vi "SimplePassRollRole.vi"(6 "Tactic index in":i32, 7 "first call":bool, 8 "error in (no error)":errorcluster, 10 "Game in":refnum<class "Game.lvclass">, 11 "SimplePassRollRole in":refnum<class "SimplePassRollRole.lvclass">) -> (0 "error out":errorcluster, 1 "tactic index":i32, 2 "Robot out":refnum<class "Robot.lvclass">, 3 "SimplePassRollRole out":refnum<class "SimplePassRollRole.lvclass">)   [LabVIEW 2023, in "SimplePassRollRole.lvclass"]
uses:
  SimplePassRollRole.lvclass
  Game_class/Game.lvclass
  Robot_class/Robot.lvclass
  Role_class/Role.lvclass/Role.ctl
  Tacticbook_class/Tacticbook.lvclass/Tacticbook.ctl
  RollerTactic_class/RollerTactic.lvclass/RollerTactic.ctl
  FollowAttackerTactic_class/FollowAttackerTactic.lvclass/FollowAttackerTactic.ctl
  PrepareRollToPassRollerGoToTactic_class/PrepareRollToPassRollerGoToTactic.lvclass/PrepareRollToPassRollerGoToTactic.ctl
  Tacticbook_class/Read RollerTactic.vi
  RollerTactic_class/Read States.vi
  Tacticbook_class/Write RollerTactic.vi
  Tacticbook_class/Read FollowAttackerTactic.vi
  FollowAttackerTactic_class/Read States.vi
  Tacticbook_class/Write FollowAttackerTactic.vi
  Tacticbook_class/Read PrepareRollToPassRollerGoToTactic.vi
  PrepareRollToPassRollerGoToTactic_class/Read States.vi
  Tacticbook_class/Write PrepareRollToPassRollerGoToTactic.vi
  Role_class/Read Tacticbook.vi
  Role_class/Write Tacticbook.vi
  Role_class/Write tactic_index.vi
  Role_class/Read RobotRef.vi
  Tacticbook_class/Tacticbook.lvclass
  RollerTactic_class/RollerTactic.lvclass
  FollowAttackerTactic_class/FollowAttackerTactic.lvclass
  PrepareRollToPassRollerGoToTactic_class/PrepareRollToPassRollerGoToTactic.lvclass
panel:
  out "Game out":refnum<class "Game.lvclass">
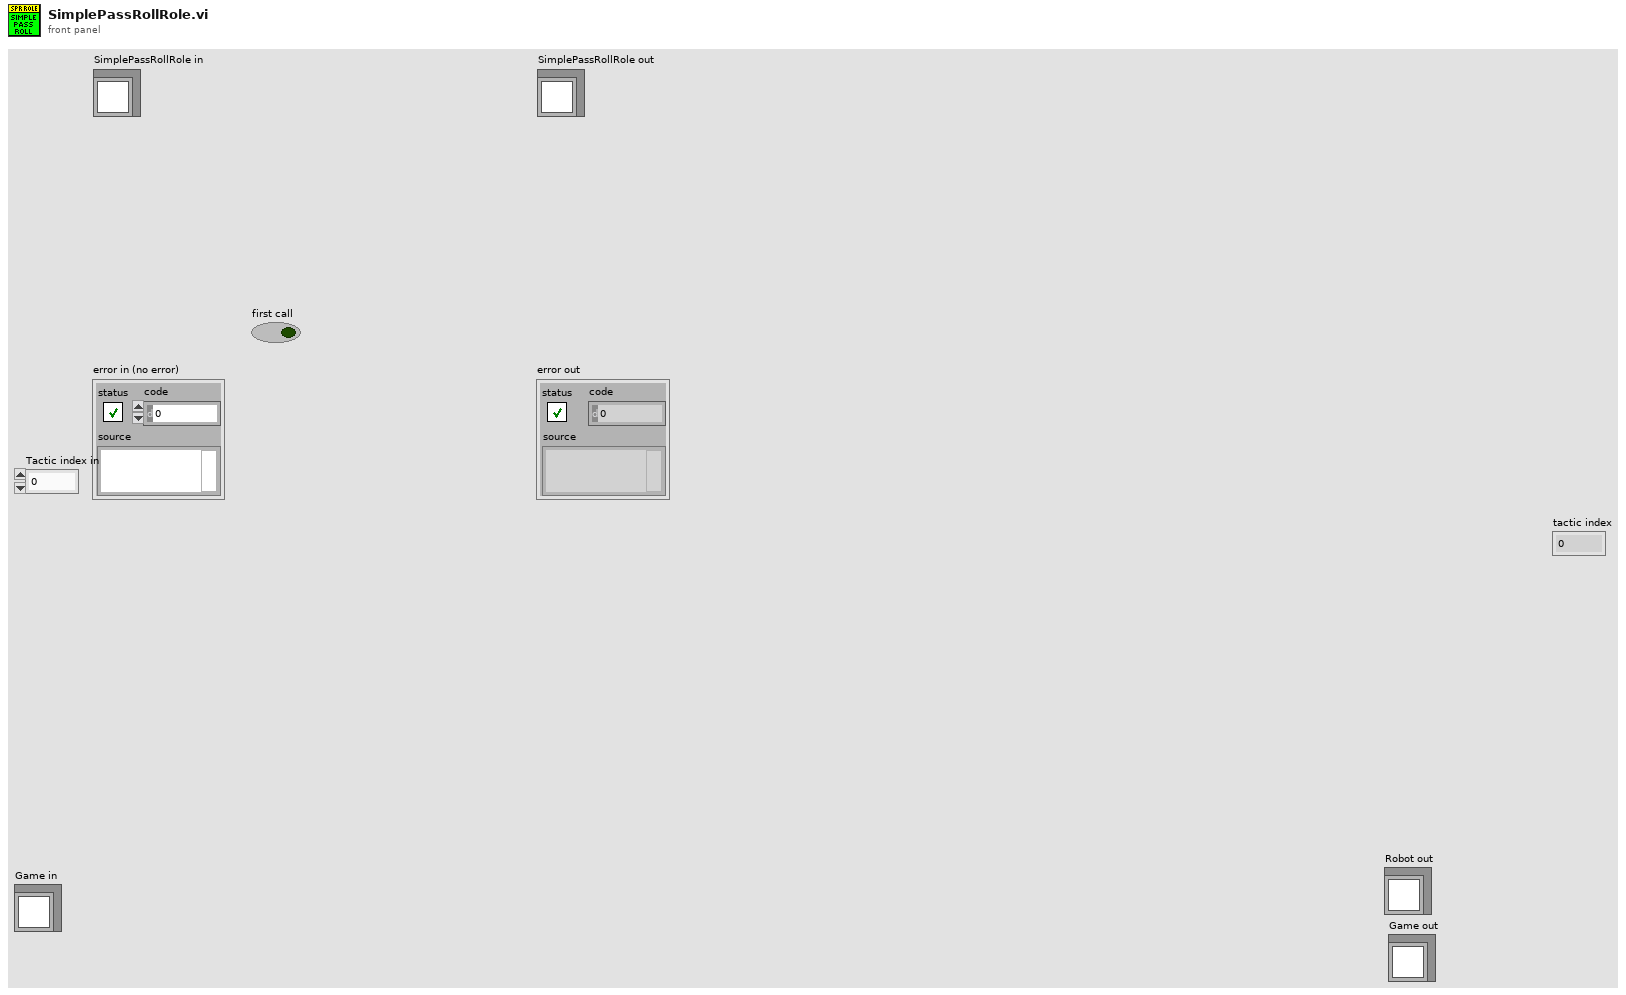
[diagram p1: front panel]
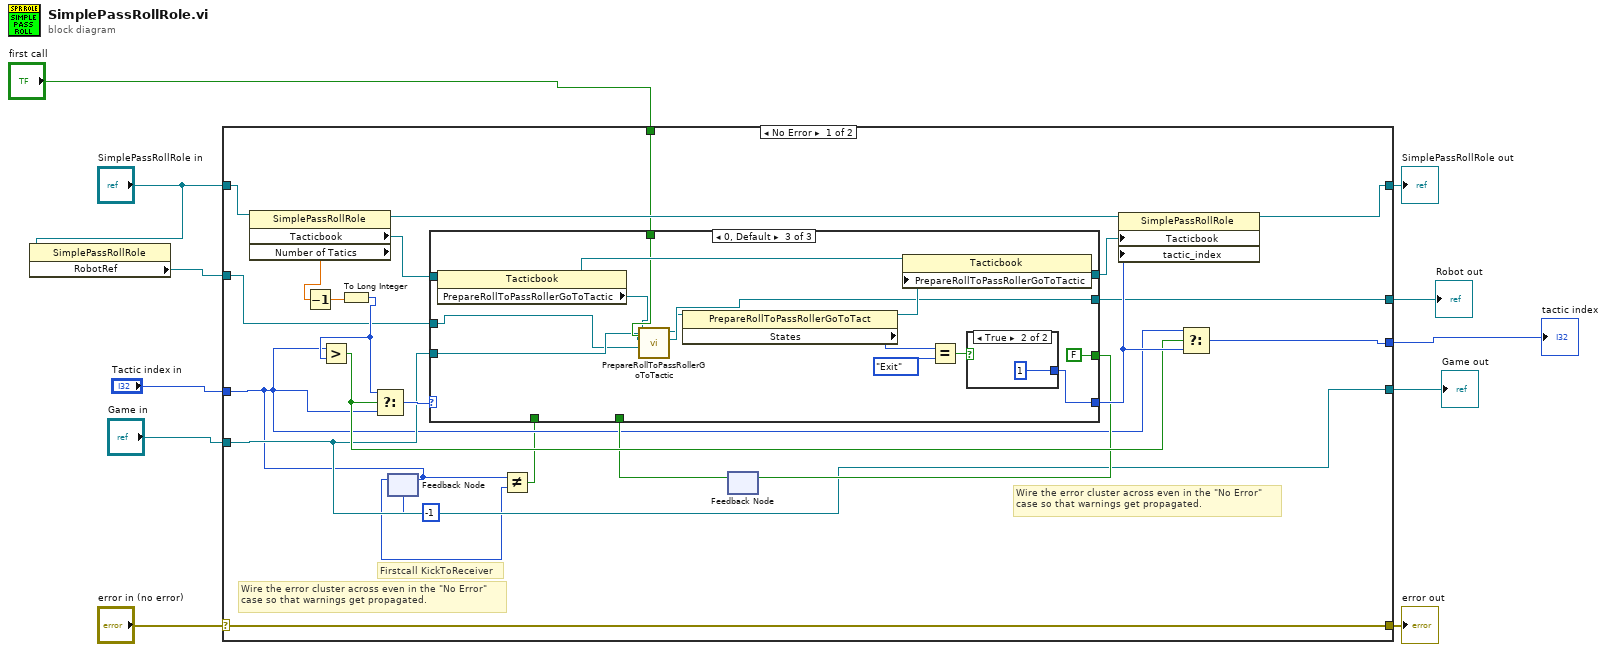
[diagram p0: block diagram]
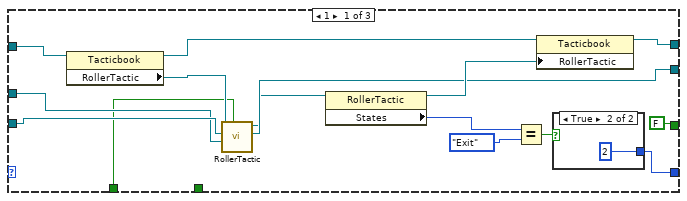
[diagram p2: hidden frame]
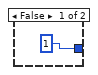
[diagram p3: hidden frame]
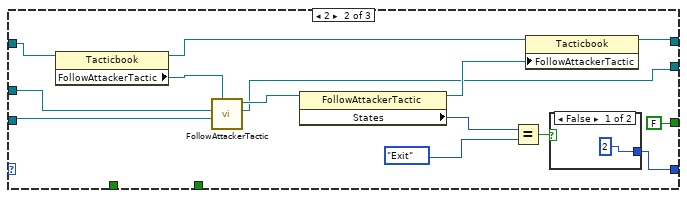
[diagram p4: hidden frame]
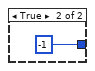
[diagram p5: hidden frame]
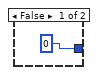
[diagram p6: hidden frame]
diagram:
  n1 = property class="SimplePassRollRole"(reference="SimplePassRollRole in") -> ("RobotRef"=w7:refnum<class "Robot.lvclass">)  [unwired: 1 in, 2 out]
  n2 = case shown="No Error" "error in (no error)" {
    selector: "error in (no error)" -> [w34 w89]
    tunnel: [w34 w89] -> w10
    tunnel: [w19 w88] -> w9
    tunnel: "SimplePassRollRole in" -> [w21 w88]
    tunnel: w7 -> [w22 w87]
    tunnel: "Tactic index in" -> [w13 w86]
    tunnel: "Game in" -> [w16 w85]
    tunnel: "first call" -> [w20 _]
    tunnel: [w18 w87] -> w3
    tunnel: [w17 w86] -> w2
    tunnel: [w16 w85] -> w1
    frame No Error {
      # "Firstcall KickToReceiver"
      # "Wire the error cluster across even in the \"No Error\"\ncase so that warnings get propagated."
      # "Wire the error cluster across even in the \"No Error\"\ncase so that warnings get propagated."
      n3 = property class="SimplePassRollRole"(reference=w21) -> (reference out=w33:refnum<class "SimplePassRollRole.lvclass">, "Tacticbook"=w32:refnum<class "Tacticbook.lvclass">, "Number of Tatics"=w27:dbl)  [unwired: 1 in, 1 out]
      n4 = Decrement(x=w27) -> (x-1=w24:dbl)
      n5 = To Long Integer(number=w24) -> (32bit integer=w23:i32)
      n6 = Greater?(x=w13, y=w23) -> (0:w28:bool)
      n7 = Select(t=w23, s=w28, f=w13) -> (s? t:f=w29:i32)
      n8 = feedback-in #1(w13) -> ()
      n9 = feedback #1(-1 ("Tactic index in")) -> (w14:i32)
      n10 = Not Equal?(x=w13, y=w14) -> (x != y?=w12:bool)
      n11 = feedback #2() -> (w25:bool)  [unwired: 1 in]
      n12 = case shown="0, Default" w29 {
        tunnel: [w43 w53 w76] -> w30
        tunnel: w32 -> [w47 w58 w82]
        tunnel: w22 -> [w39 w57 w71]
        tunnel: [w38 w55 w70] -> w18
        tunnel: [w45 w54 w79] -> w31
        tunnel: w16 -> [w40 w56 w72]
        tunnel: w20 -> [_ _ w74]
        tunnel: [FALSE FALSE FALSE] -> w26
        tunnel: w25 -> [_ _ _]
        tunnel: w12 -> [w36 _ _]
        frame 1 {
          n13 = property class="Tacticbook"(reference=w47) -> (reference out=w46:refnum<class "Tacticbook.lvclass">, "RollerTactic"=w41:refnum<class "RollerTactic.lvclass">)  [unwired: 1 in, 1 out]
          n14 = call "RollerTactic.vi"("first call"=w36, "Robot"=w39, "Game in"=w40, "RollerTactic in"=w41) -> ("Robot out"=w38:refnum<class "Robot.lvclass">, "RollerTactic out"=w37:refnum<class "RollerTactic.lvclass">)  [unwired: 5 in, 1 out]
          n15 = property class="RollerTactic"(reference=w37) -> (reference out=w44:refnum<class "RollerTactic.lvclass">, "States"=w48:enum16{"Exit", "Roller"})  [unwired: 1 in, 1 out]
          n16 = Equal?(x=w48, y=enum16{"Exit", "Roller"}."Exit") -> (x = y?=w49:bool)
          n17 = property class="Tacticbook"(reference=w46, "RollerTactic"=w44) -> (reference out=w45:refnum<class "Tacticbook.lvclass">)  [unwired: 1 in, 1 out]
          n18 = case shown="True" w49 {
            tunnel: [1 2] -> w43
            frame False {
            }
            frame True {
            }
          }
        }
        frame 2 {
          n19 = property class="Tacticbook"(reference=w58) -> (reference out=w63:refnum<class "Tacticbook.lvclass">, "FollowAttackerTactic"=w61:refnum<class "FollowAttackerTactic.lvclass">)  [unwired: 1 in, 1 out]
          n20 = call-dynamic "FollowAttackerTactic.vi"("Game in"=w56, "Robot"=w57, "FollowAttackerTactic in"=w61) -> ("Robot out"=w55:refnum<class "Robot.lvclass">, "FollowAttackerTactic out"=w60:refnum<class "FollowAttackerTactic.lvclass">)  [unwired: 6 in, 1 out]
          n21 = property class="FollowAttackerTactic"(reference=w60) -> (reference out=w62:refnum<class "FollowAttackerTactic.lvclass">, "States"=w64:enum16{"Exit", "FollowAttacker"})  [unwired: 1 in, 1 out]
          n22 = Equal?(x=w64, y=enum16{"Exit", "FollowAttacker"}."Exit" ("States")) -> (x = y?=w65:bool)
          n23 = property class="Tacticbook"(reference=w63, "FollowAttackerTactic"=w62) -> (reference out=w54:refnum<class "Tacticbook.lvclass">)  [unwired: 1 in, 1 out]
          n24 = case shown="False" w65 {
            tunnel: [2 -1] -> w53
            frame False {
            }
            frame True {
            }
          }
        }
        frame 0, Default {
          n25 = property class="Tacticbook"(reference=w82) -> (reference out=w81:refnum<class "Tacticbook.lvclass">, "PrepareRollToPassRollerGoToTactic"=w73:refnum<class "PrepareRollToPassRollerGoToTactic.lvclass">)  [unwired: 1 in, 1 out]
          n26 = call "PrepareRollToPassRollerGoToTactic.vi"("first call"=w74, "Robot"=w71, "Game in"=w72, "PrepareRollToPassRollerGoToTactic in"=w73) -> ("Robot out"=w70:refnum<class "Robot.lvclass">, "PrepareRollToPassRollerGoToTactic out"=w69:refnum<class "PrepareRollToPassRollerGoToTactic.lvclass">)  [unwired: 5 in, 1 out]
          n27 = property class="PrepareRollToPassRollerGoToTact"(reference=w69) -> (reference out=w80:refnum<class "PrepareRollToPassRollerGoToTactic.lvclass">, "States"=w77:enum16{"GoTo", "Exit"})  [unwired: 1 in, 1 out]
          n28 = property class="Tacticbook"(reference=w81, "PrepareRollToPassRollerGoToTactic"=w80) -> (reference out=w79:refnum<class "Tacticbook.lvclass">)  [unwired: 1 in, 1 out]
          n29 = Equal?(x=w77, y=enum16{"GoTo", "Exit"}."Exit") -> (x = y?=w78:bool)
          n30 = case shown="True" w78 {
            tunnel: [0 1] -> w76
            frame False {
            }
            frame True {
            }
          }
        }
      }
      n31 = feedback-in #2(w26) -> ()
      n32 = property class="SimplePassRollRole"(reference=w33, "Tacticbook"=w31, "tactic_index"=w30) -> (reference out=w19:refnum<class "SimplePassRollRole.lvclass">)  [unwired: 1 in, 1 out]
      n33 = Select(t=w13, s=w28, f=w30) -> (s? t:f=w17:i32)
    }
    frame Error {
    }
  }
  "error out" <- w10
  "SimplePassRollRole out" <- w9
  "Robot out" <- w3
  "Game out" <- w1
  "tactic index" <- w2
